vi "Write-U64-for-UART.vi"(10 "Log Message":string="DBG-READ", 11 "Data":u64[](array[numeric])=[1234605616436508552, 11578966645329104914] format="%.0x") -> (3 "concatenated string":string)   [LabVIEW 2018]
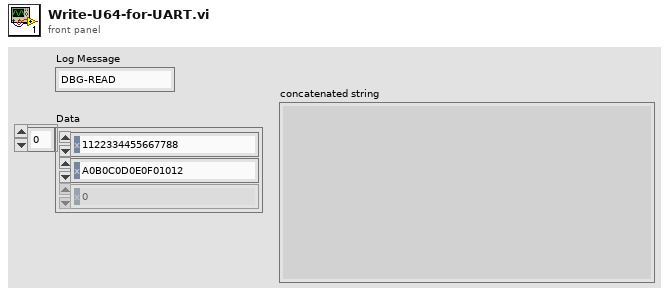
[diagram p1: front panel]
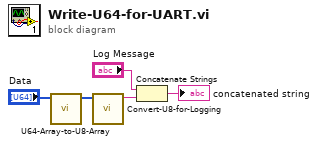
[diagram p0: block diagram]
diagram:
  n1 = call "U64-Array-to-U8-Array.vi"("U64 [] in"="Data") -> ("U8 [] out"=w2:u8[])  [unwired: 10 in]
  n2 = call "Convert-U8-for-Logging.vi"("u8 Array"=w2) -> ("Output String"=w3:string)  [unwired: 10 in]
  n3 = Concatenate Strings("Log Message", w3) -> (→"concatenated string":string)
